vi "avoidPotentialFieldBlockRobot.vi"(8 "error in (no error)":errorcluster, 9 "multiplier":dbl, 10 "potentialFieldVelocities":dbl[](array[numeric]), 11 "Robot in":refnum<class "Robot.lvclass">) -> (0 "error out":errorcluster, 2 "v_tang/v_norm":dbl[](array[numeric]), 3 "Robot out":refnum<class "Robot.lvclass">)   [LabVIEW 2023, in "Robot.lvclass"]
uses:
  Robot.lvclass
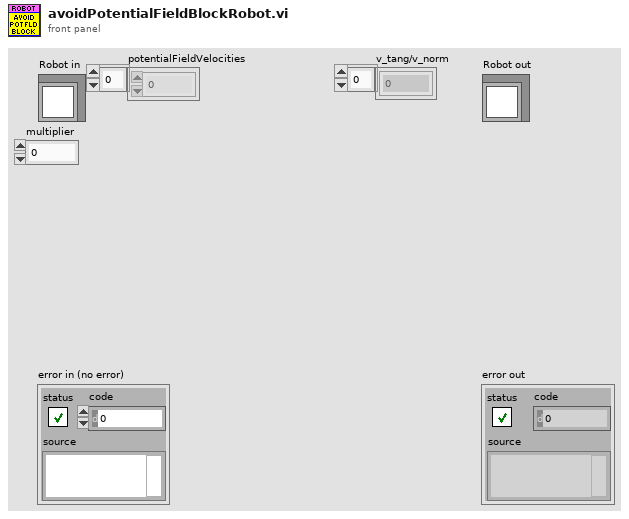
[diagram p1: front panel]
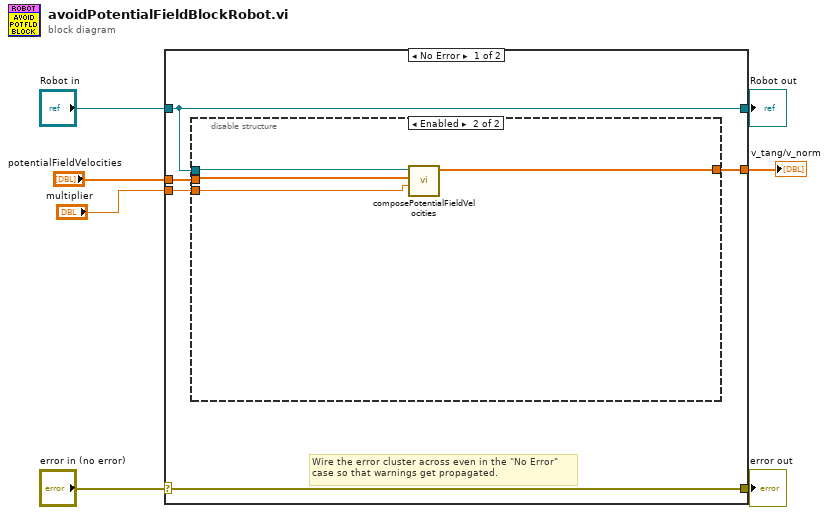
[diagram p0: block diagram]
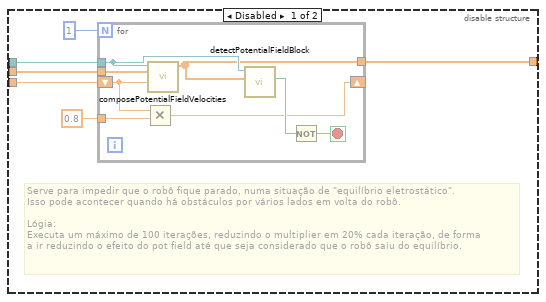
[diagram p2: hidden frame]
diagram:
  n1 = case shown="No Error" "error in (no error)" {
    selector: "error in (no error)" -> [w12 w32]
    tunnel: [w12 w32] -> w6
    tunnel: [w9 w31] -> w4
    tunnel: "Robot in" -> [w9 w31]
    tunnel: "potentialFieldVelocities" -> [w10 _]
    tunnel: "multiplier" -> [w11 _]
    tunnel: [w8 _] -> w1
    frame No Error {
      # "Wire the error cluster across even in the \"No Error\"\ncase so that warnings get propagated."
      n2 = disable-structure shown="Enabled" {
        disable-tunnel: w11 -> [w17 w27]
        disable-tunnel: w10 -> [w16 w28]
        disable-tunnel: w9 -> [w15 w29]
        disable-tunnel: [w13 w30] -> w8
        frame Disabled {
          # "Serve para impedir que o robô fique parado, numa situação de \"equilíbrio eletrostático\".\nIsso pode acontecer quando há obstáculos por vários lados em volta do robô.\n\nLógia:\nExecuta um máximo de 100 iterações, reduzindo o multiplier em 20% cada iteração, de forma\na ir reduzindo o efeito do pot field até que seja considerado que o robô saiu do equilíbrio."
          n3 = for {
            N: 1 -> [_]
            tunnel: w16 -> [w24]
            tunnel: w15 -> [w20]
            shift-right: [w21] -> _
            shift-left: w17 -> [w23]
            tunnel: 0.8 ("y") -> [w22]
            tunnel: [w19] -> w13
            stop <- w26 stop-if-true
            n4 = Multiply(x=w23, y=w22) -> (x*y=w21:dbl)
            n5 = call "composePotentialFieldVelocities.vi"("multiplier"=w23, "potentialFieldVelocities"=w24, "Robot in"=w20) -> ("v_tang/v_norm"=w19:dbl[])  [unwired: 8 in]
            n6 = call "detectPotentialFieldBlock.vi"("v_tang/v_norm resultant"=w19, "Robot in"=w20) -> ("potentialFieldBlockedRobot"=w25:bool)  [unwired: 7 in, 2 out]
            n7 = Not(x=w25) -> (.not. x?=w26:bool)
          }
        }
        frame Enabled {
          n8 = call "composePotentialFieldVelocities.vi"("multiplier"=w27, "potentialFieldVelocities"=w28, "Robot in"=w29) -> ("v_tang/v_norm"=w30:dbl[])  [unwired: 8 in]
        }
      }
    }
    frame Error {
    }
  }
  "error out" <- w6
  "Robot out" <- w4
  "v_tang/v_norm" <- w1
